vi "Save.vi"(0 "User Manager View in":refnum<class "User Manager View.lvclass">, 11 "error in (no error)":errorcluster) -> (4 "User Manager View out":refnum<class "User Manager View.lvclass">, 15 "error out":errorcluster)   [LabVIEW 2017, in "User Manager View.lvlib" / "User Manager View.lvclass"]
uses:
  <vilib>/gpm_packages/@cs/User Manager App/User Manager View/User Manager View/User Manager View.lvclass
  <vilib>/gpm_packages/@cs/User Manager App/User Manager Model/Type Definitions/New User Information.ctl
  <vilib>/gpm_packages/@cs/User Manager App/User Manager Model/Type Definitions/Credentials.ctl
  <vilib>/gpm_packages/@cs/User Manager App/User Manager Model/Type Definitions/User Levels.ctl
  <vilib>/gpm_packages/@cs/User Manager App/User Manager View/User Manager View/User Manager View.lvclass/User Manager View.ctl
  <vilib>/gpm_packages/@cs/User Manager App/User Manager Model/Type Definitions/User Manager Application Types.lvlib
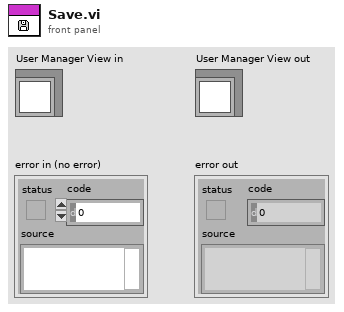
[diagram p1: front panel]
types:
  T1 = typedef "User Manager Application Types.lvlib/New User Information.ctl" = cluster{"User Info":T2, "User Level":T3}
  T2 = typedef "User Manager Application Types.lvlib/Credentials.ctl" = cluster{"Username":string, "Password":string}
  T3 = typedef "User Manager Application Types.lvlib/User Levels.ctl" = cluster{"Rank":i32, "Title":string}
  T4 = enum8{"Enabled", "Disabled", "Disabled and Grayed Out"}
  T5 = typedef "User Manager View.lvlib/State.ctl" = enum16{"Normal", "Adding User", "Changing User Data"}
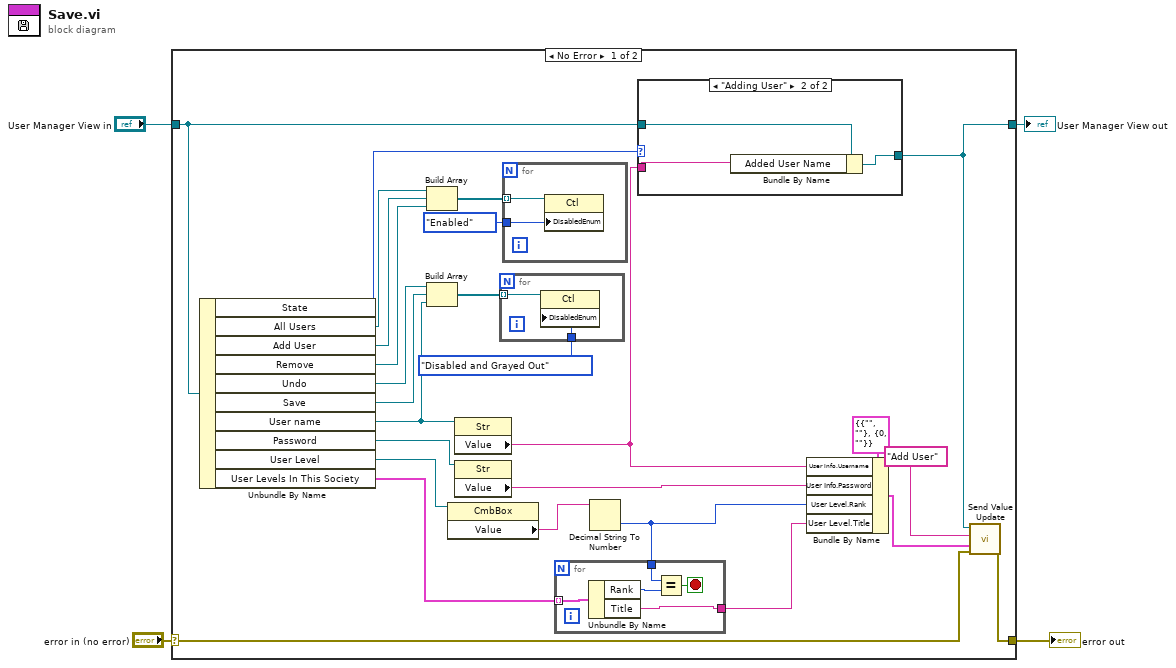
[diagram p0: block diagram]
diagram:
  n1 = case shown="No Error" "error in (no error)" {
    selector: "error in (no error)" -> [w23 w45]
    tunnel: [w22 w45] -> w3
    tunnel: [w20 w44] -> w1
    tunnel: "User Manager View in" -> [w21 w44]
    frame No Error {
      n2 = Unbundle By Name(w21) -> ("State"=w8:T5, "All Users"=w9:refnum<vi>, "Add User"=w10:refnum<vi>, "Remove"=w11:refnum<vi>, "Undo"=w12:refnum<vi>, "Save"=w13:refnum<vi>, "User name"=w14:refnum<vi>, "Password"=w26:refnum<vi>, "User Level"=w29:refnum<vi>, "User Levels In This Society"=w27:T3[])
      n3 = Build Array(w9, w10, w11) -> (w19:refnum<vi>[])
      n4 = Build Array(w12, w13, w14) -> (w16:refnum<vi>[])
      n5 = property class="CmbBox"(reference=w29) -> ("Value"=w24:string)  [unwired: 1 in, 2 out]
      n6 = property class="Str"(reference=w14) -> ("Value"=w15:string)  [unwired: 1 in, 2 out]
      n7 = property class="Str"(reference=w26) -> ("Value"=w25:string)  [unwired: 1 in, 2 out]
      n8 = for {
        tunnel: w16 -> [w36] mode=indexing
        tunnel: T4."Disabled and Grayed Out" ("Disabled") -> [w35]
        n9 = property class="Ctl"(reference=w36, "DisabledEnum"=w35) -> ()  [unwired: 1 in, 2 out]
      }
      n10 = for {
        tunnel: w19 -> [w38] mode=indexing
        tunnel: T4."Enabled" ("Disabled") -> [w37]
        n11 = property class="Ctl"(reference=w38, "DisabledEnum"=w37) -> ()  [unwired: 1 in, 2 out]
      }
      n12 = Decimal String To Number(string=w24) -> (number=w6:i32)  [unwired: 2 in, 1 out]
      n13 = for {
        tunnel: w27 -> [w43] mode=indexing
        tunnel: [w41] -> w7
        tunnel: w6 -> [w40]
        stop <- w42 stop-if-true
        n14 = Unbundle By Name(w43) -> ("Rank"=w39:i32, "Title"=w41:string)
        n15 = Equal?(x=w40, y=w39) -> (x = y?=w42:bool)
      }
      n16 = case shown="\"Adding User\"" w8 {
        tunnel: w21 -> [w31 w34]
        tunnel: [w31 w33] -> w20
        tunnel: w15 -> [_ w32]
        frame "Normal", Default {
        }
        frame "Adding User" {
          n17 = Bundle By Name(cluster=w34, "Added User Name"=w32) -> (w33:refnum<class "User Manager View.lvclass">)
        }
      }
      n18 = Bundle By Name(cluster=T1 {"User Info"={"Username"="", "Password"=""}, "User Level"={"Rank"=0, "Title"=""}} ("New Uer Info"), "User Info.Username"=w15, "User Info.Password"=w25, "User Level.Rank"=w6, "User Level.Title"=w7) -> (w28:T1)
      n19 = call-dynamic "Send Value Update.vi"("error in (no error)"=w23, "Value"=w28, "Datum Name"="Add User", "IViewable in"=w20) -> ("error out"=w22:errorcluster)  [unwired: 7 in]
    }
    frame Error {
    }
  }
  "error out" <- w3
  "User Manager View out" <- w1
